vi "Read BuildSpec Map.vi"(8 "error in (no error)":errorcluster, 11 "LabVIEW Build Script in":refnum<class "LabVIEW Build Script.lvclass">) -> (0 "error out":errorcluster, 2 "BuildSpec Map":T1, 3 "LabVIEW Build Script out":refnum<class "LabVIEW Build Script.lvclass">)   [LabVIEW 2021, in "LabVIEW Build Script.lvclass"]
uses:
  LabVIEW Build Script.lvclass
  LabVIEW Build Script.lvclass/LabVIEW Build Script.ctl
  <vilib>/CIF Foundation/CIF LabVIEW Scripting/LV Scripting/Typedef/BuildSpec Map.ctl
  <vilib>/CIF Foundation/CIF LabVIEW Scripting/LV Scripting/LV Scripting Utilities.lvlib
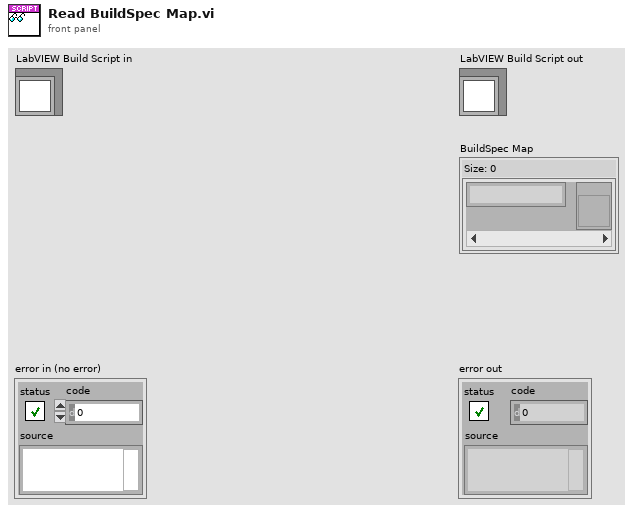
[diagram p1: front panel]
types:
  T1 = typedef "LV Scripting Utilities.lvlib/BuildSpec Map.ctl" = map{string, refnum<vi>}
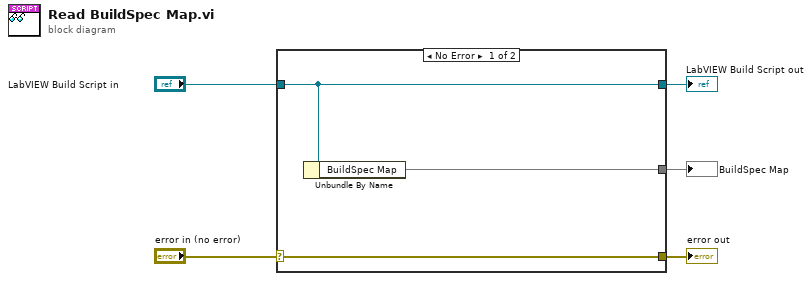
[diagram p0: block diagram]
diagram:
  n1 = case shown="No Error" "error in (no error)" {
    selector: "error in (no error)" -> [w8 w9]
    tunnel: [w8 w9] -> w4
    tunnel: [w7 w10] -> w2
    tunnel: "LabVIEW Build Script in" -> [w7 w10]
    tunnel: [w6 _] -> w1
    frame No Error {
      n2 = Unbundle By Name(w7) -> ("BuildSpec Map"=w6:T1)
    }
    frame Error {
    }
  }
  "error out" <- w4
  "LabVIEW Build Script out" <- w2
  "BuildSpec Map" <- w1
